vi "Core Destroy.vi"(8 "error in (no error)":errorcluster, 11 "CIFTemplateNode in":refnum<class "CIFTemplateNode.lvclass">) -> (0 "error out":errorcluster, 3 "CIFTemplateNode out":refnum<class "CIFTemplateNode.lvclass">)   [LabVIEW 2021, in "CIFTemplateNode.lvclass"]
uses:
  CIFTemplateNode.lvclass
  CIFTemplateNode.lvclass/CIFTemplateNode.ctl
  CIFUtilities/CIFOutOfBand/CIFOutOfBand.lvclass
  CIFTemplateGrpc/CIF_Plugin_Core_server/RPC Service/PluginCore/PluginCore.lvclass
  CIFTemplateCoreOOB/OOB_Rx/CIFTemplateCoreOOB_Rx.lvclass
  CIFTemplateCoreOOB/OOB_Tx/CIFTemplateCoreOOB_Tx.lvclass
  D:/dev/CIF-LVCore/src/CIFUtilities/CIFOutOfBand/CIFOutOfBand.lvclass
  D:/dev/CIF-LVCore/src/CIFTemplate/CIFTemplateCoreOOB/OOB_Rx/CIFTemplateCoreOOB_Rx.lvclass
  D:/dev/CIF-LVCore/src/CIFTemplate/CIFTemplateCoreOOB/OOB_Tx/CIFTemplateCoreOOB_Tx.lvclass
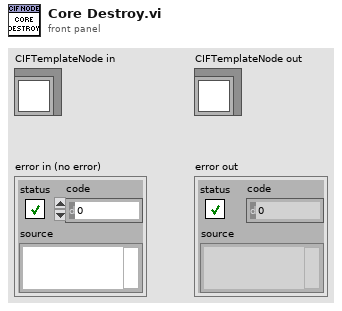
[diagram p1: front panel]
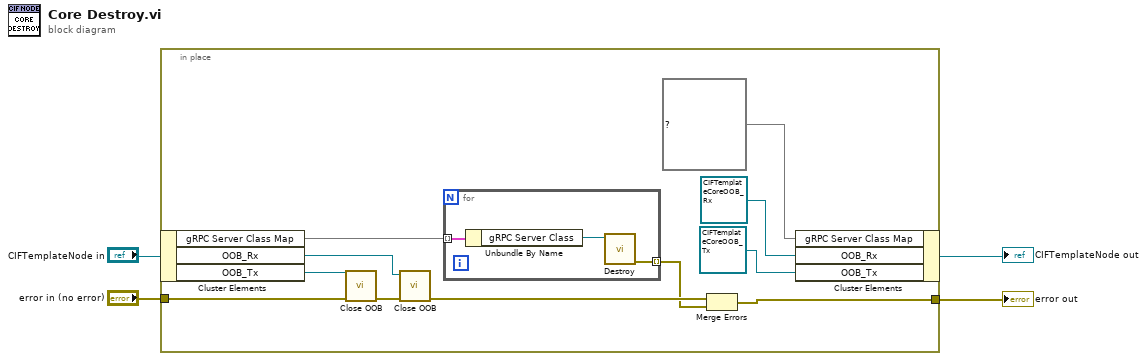
[diagram p0: block diagram]
diagram:
  n1 = in-place {
    in-place-border: "error in (no error)" -> [w15]
    in-place-border: [w8] -> w3
    n2 = in-place-cluster #1("CIFTemplateNode in") -> ("gRPC Server Class Map"=w11:map{string, refnum<class "PluginCore.lvclass">}, "OOB_Rx"=w13:refnum<class "CIFTemplateCoreOOB_Rx.lvclass">, "OOB_Tx"=w12:refnum<class "CIFTemplateCoreOOB_Tx.lvclass">)
    n3 = call "Close OOB.vi"("error in"=w15, "OOB in"=w12) -> ("error out"=w14:errorcluster)  [unwired: 9 in]
    n4 = call "Close OOB.vi"("error in"=w14, "OOB in"=w13) -> ("error out"=w10:errorcluster)  [unwired: 9 in]
    n5 = for {
      tunnel: w11 -> [w18] mode=indexing
      tunnel: [w16] -> w9 mode=indexing
      n6 = Unbundle By Name(w18) -> ("gRPC Server Class"=w17:refnum<class "PluginCore.lvclass">)
      n7 = call-dynamic "Destroy.vi"("SignalGeneratorService in"=w17) -> ("error out"=w16:errorcluster)  [unwired: 9 in, 1 out]
    }
    n8 = Merge Errors(w10, w9) -> (w8:errorcluster)
    n9 = in-place-cluster #1("gRPC Server Class Map"=map{string, refnum<class "PluginCore.lvclass">} {}, "OOB_Rx"=refnum<class "CIFTemplateCoreOOB_Rx.lvclass"> refnum, "OOB_Tx"=refnum<class "CIFTemplateCoreOOB_Tx.lvclass"> refnum) -> (→"CIFTemplateNode out":refnum<class "CIFTemplateNode.lvclass">)
  }
  "error out" <- w3
